vi "Target.vi"() -> ()   [LabVIEW 2013]
uses:
  shared/iRobot Sensor Display.ctl
  Statechart.lvsc/StatechartState.ctl
  Statechart.lvsc/State.ctl
  shared/Sensors.ctl
  iRobot/Sensor/Accelerometer.ctl
  iRobot/Sensor/Sensor Group 6.ctl
  iRobot/Sensor/Bumps + Wheel Drops.ctl
  iRobot/Sensor/Buttons.ctl
  iRobot/Sensor/Charging State.ctl
  iRobot/Sensor/Charging Sources Available.ctl
  iRobot/Sensor/OI Mode.ctl
  iRobot/Sensor/Cargo Bay Digital Inputs.ctl
  iRobot/Sensor/Low-Side Driver + Wheel Overcurrent.ctl
  Statechart.lvsc/CompanionDiagram.vi/42/SC Main.vi
  Statechart.lvsc/CompanionDiagram.vi/42/Upd State.vi
  Statechart.lvsc/CompanionDiagram.vi/42/Trans Graph0.vi
  Statechart.lvsc/CompanionDiagram.vi/42/EnterGraphCore.vi
  <vilib>/myRIO/Common/Instrument Driver Framework/myRIO v1.0/UART/vis/myRIO v1.0 Close UART.vi
  Statechart.lvsc/CompanionDiagram.vi/42/Trans Graph1.vi
  Statechart.lvsc/CompanionDiagram.vi/42/Trans Graph2.vi
  <vilib>/myRIO/Common/Instrument Driver Framework/myRIO v1.0/myRIO v1.1 Open.vi
  Statechart.lvsc/CompanionDiagram.vi
  shared/Wrap Angle.vi
  <vilib>/myRIO/Common/Instrument Driver Framework/Utilities/vis/FPGA Ref Manager.vi
  <vilib>/myRIO/Common/Instrument Driver Framework/myRIO v1.0/myRIO v1.0 Reset FPGA.vi
  Statechart.lvsc/Trigger.ctl
  <vilib>/Statechart/Infrastructure/RTStatechart/RunTime SCN.xnode
  Statechart.lvsc/Inputs.ctl
  Statechart.lvsc/Outputs.ctl
  Statechart.lvsc
  <vilib>/myRIO/Instrument Drivers/Utilities/Utilities.lvlib
panel:
  in  "Tab Control":T1(tab)
  out "iRobot Sensors (graphical)":T2 {"Right Wheel (mm/s)" scale=-500.0..500.0; "Left Wheel (mm/s)" scale=-500.0..500.0}
  out "Active States":T4
  out "error out":errorcluster
  in  "stop":bool
  out "Target Running":bool
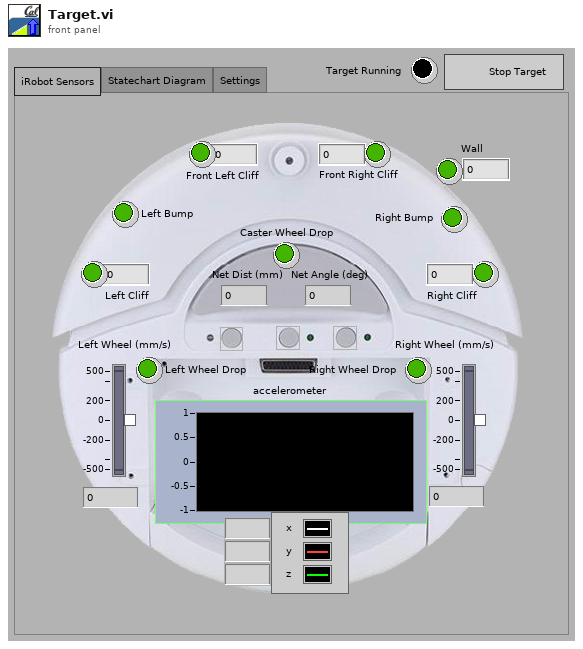
[diagram p1: front panel]
types:
  T1 = enum32{"iRobot Sensors", "Statechart Diagram", "Settings"}
  T2 = typedef "iRobot Sensor Display.ctl" = cluster{"Caster Wheel Drop":bool, "Left Wheel Drop":bool, "Right Wheel Drop":bool, "Left Bump":bool, "Right Bump":bool, "Left Cliff":bool, "Front Left Cliff":bool, "Front Right Cliff":bool, "Right Cliff":bool, "Wall":bool, "Net Dist (mm)":i32, "Net Angle (deg)":i32, "Wall":u16, "Left Cliff":u16, "Front Left Cliff":u16, "Front Right Cliff":u16, "Right Cliff":u16, "Left Wheel (mm/s)":i16, "Right Wheel (mm/s)":i16, "accelerometer":T3}
  T3 = typedef "Accelerometer.ctl" = cluster{"x axis (g)":dbl, "y axis (g)":dbl, "z axis (g)":dbl}
  T4 = typedef "Statechart.lvsc/StatechartState.ctl" = T5[]
  T5 = typedef "Statechart.lvsc/State.ctl" = enum16{"NI.SC.Initial", "NI.SC.History", "NI.SC.ShallowHistory", "NI.SC.Terminal", "Pause", "Run", "Pause\\Detect Play Button\\Pause;\nWait for\nbutton\nrelease", "Pause\\Detect Play Button\\Unpause;\nwait for\nbutton release", "Pause\\Detect Play Button\\Unpause;\nwait for\nbutton press", "Run\\Run Mode\\Turn", "Run\\Run Mode\\Drive"}
  T6 = typedef "iRobot UART Port Type.ctl" = refnum<visa-resource-name>
  T7 = typedef "Sensors.ctl" = cluster{"net distance (mm)":i32, "net angle (deg)":i32, "accelerometer":T3, "iRobot Sensors":T8, "Is Simulator?":bool}
  T8 = typedef "Sensor Group 6.ctl" = cluster{"Bumps + Wheel Drops":T9, "Wall":bool, "Cliff Left":bool, "Cliff Front Left":bool, "Cliff Front Right":bool, "Cliff Right":bool, "Wall Signal":u16, "Cliff Left Signal":u16, "Cliff Front Left Signal":u16, "Cliff Front Right Signal":u16, "Cliff Right Signal":u16, "Buttons":T10, "Virtual Wall":bool, "# Stream Packets":u8, "Requested Velocity (mm/s)":i16, "Requested Radius (mm)":i16, "Requested Right Wheel Velocity (mm/s)":i16, "Requested Left Wheel Velocity (mm/s)":i16, "Distance (mm)":i32, "Angle (deg)":i32, "Song Playing":bool, "Song Number":u8, "Charging State":T11, "Voltage (mV)":u16, "Current (mA)":i16, "Battery Temperature (deg C)":i8, "Battery Charge (mAh)":u16, "Battery Capacity (mAh)":u16, "Charging Sources":T12, "OI Mode":T13, "Digital Inputs":T14, "Drivers & Wheel Overcurrent":T15, "Analog Signal":u16, "Infrared":u8}
  T9 = typedef "Bumps + Wheel Drops.ctl" = cluster{"Wheeldrop Caster":bool, "Wheeldrop Left":bool, "Wheeldrop Right":bool, "Bump Left":bool, "Bump Right":bool}
  T10 = typedef "Buttons.ctl" = cluster{"Advance":bool, "Play":bool}
  T11 = typedef "Charging State.ctl" = enum16{"Not Charging", "Reconditioning Charging", "Full Charging", "Trickle Charging", "Waiting", "Charging Fault Condition"}
  T12 = typedef "Charging Sources Available.ctl" = cluster{"Internal Charger":bool, "Home Base":bool}
  T13 = typedef "OI Mode.ctl" = enum16{"Off", "Passive", "Safe", "Full"}
  T14 = typedef "Cargo Bay Digital Inputs.ctl" = cluster{"Digital Input 0":bool, "Digital Input 1":bool, "Digital Input 2":bool, "Digital Input 3":bool, "Device Detect":bool}
  T15 = typedef "Low-Side Driver + Wheel Overcurrent.ctl" = cluster{"Low-Side Driver 0":bool, "Low-Side Driver 1":bool, "Low-Side Driver 2":bool, "Left Wheel":bool, "Right Wheel":bool}
  T16 = typedef "Statechart.lvsc/Outputs.ctl" = cluster{"Left Wheel Speed (mm/s)":i16, "Right Wheel Speed (mm/s)":i16}
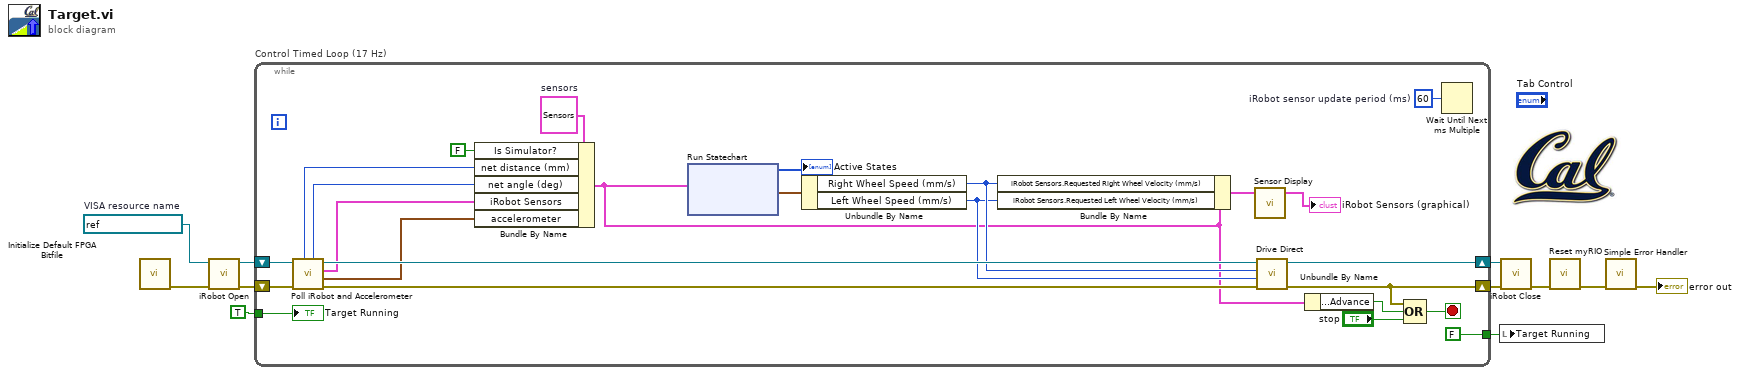
[diagram p0: block diagram]
diagram:
  w5 = refnum<visa-resource-name> "ASRL1::INSTR"  # VISA resource name
  n1 = call <vilib>:"Initialize Default FPGA Bitfile.vi"() -> ("error out"=w3:errorcluster)  [unwired: 11 in]
  n2 = call "iRobot Open.vi"("error in (no error)"=w3, "UART port in"=w5) -> ("error out"=w10:errorcluster, "UART port out"=w9:T6)  [unwired: 8 in]
  n3 = while "Control Timed Loop (17 Hz)" {
    shift-right: [w36] -> w11
    shift-left: w9 -> [w32]
    shift-right: [w16] -> w6
    shift-left: w10 -> [w31]
    tunnel: TRUE ("stop") -> [w26]
    tunnel: [FALSE ("stop")] -> w7
    stop <- w35 stop-if-true
    w18 = T7 {"net distance (mm)"=0, "net angle (deg)"=0, "accelerometer"={"x axis (g)"=0.0, "y axis (g)"=0.0, "z axis (g)"=0.0}, "iRobot Sensors"={"Bumps + Wheel Drops"={"Wheeldrop Caster"=FALSE, "Wheeldrop Left"=FALSE, "Wheeldrop Right"=FALSE, "Bump Left"=FALSE, "Bump Right"=FALSE}, "Wall"=FALSE, "Cliff Left"=FALSE, "Cliff Front Left"=FALSE, "Cliff Front Right"=FALSE, "Cliff Right"=FALSE, "Wall Signal"=0, "Cliff Left Signal"=0, "Cliff Front Left Signal"=0, "Cliff Front Right Signal"=0, "Cliff Right Signal"=0, "Buttons"={"Advance"=FALSE, "Play"=FALSE}, "Virtual Wall"=FALSE, "# Stream Packets"=0, "Requested Velocity (mm/s)"=0, "Requested Radius (mm)"=0, "Requested Right Wheel Velocity (mm/s)"=0, "Requested Left Wheel Velocity (mm/s)"=0, "Distance (mm)"=0, "Angle (deg)"=0, "Song Playing"=FALSE, "Song Number"=0, "Charging State"=enum."Not Charging", "Voltage (mV)"=0, "Current (mA)"=0, "Battery Temperature (deg C)"=0, "Battery Charge (mAh)"=0, "Battery Capacity (mAh)"=0, "Charging Sources"={"Internal Charger"=FALSE, "Home Base"=FALSE}, "OI Mode"=enum."Off", "Digital Inputs"={"Digital Input 0"=FALSE, "Digital Input 1"=FALSE, "Digital Input 2"=FALSE, "Digital Input 3"=FALSE, "Device Detect"=FALSE}, "Drivers & Wheel Overcurrent"={"Low-Side Driver 0"=FALSE, "Low-Side Driver 1"=FALSE, "Low-Side Driver 2"=FALSE, "Left Wheel"=FALSE, "Right Wheel"=FALSE}, "Analog Signal"=0, "Infrared"=255}, "Is Simulator?"=FALSE}  # sensors
    w20 = u32 60  # iRobot sensor update period (ms)
    n4 = call "Poll iRobot and Accelerometer.vi"("error in"=w31, "UART port in"=w32) -> ("error out"=w30:errorcluster, "Acceleration (g)"=w21:T3, "iRobot SensorGroup6"=w24:T8, "UART port out"=w29:T6, "net angle (deg)"=w27:i32, "net distance (mm)"=w28:i32)  [unwired: 4 in]
    n5 = Bundle By Name(cluster=w18, "Is Simulator?"=FALSE, "net distance (mm)"=w28, "net angle (deg)"=w27, "iRobot Sensors"=w24, "accelerometer"=w21) -> (w12:T7)
    n6 = xnode "Run Statechart"("Inputs"=w12) -> ("Outputs"=w34:T16, "Active States"=→"Active States":T4)  [unwired: 2 in, 1 out]
    n7 = Unbundle By Name(w34) -> ("Right Wheel Speed (mm/s)"=w15:i16, "Left Wheel Speed (mm/s)"=w14:i16)
    n8 = Bundle By Name(cluster=w12, "iRobot Sensors.Requested Right Wheel Velocity (mm/s)"=w15, "iRobot Sensors.Requested Left Wheel Velocity (mm/s)"=w14) -> (w13:T7)
    n9 = call "Sensor Display.vi"("sensors"=w13) -> ("irobot sensor display"=→"iRobot Sensors (graphical)":T2)  [unwired: 4 in]
    n10 = call "Drive Direct.vi"("error in"=w30, "Left Wheel Velocity (mm/s)"=w14, "Right Wheel Velocity (mm/s)"=w15, "UART port in"=w29) -> ("error out"=w16:errorcluster, "UART port out"=w36:T6)  [unwired: 6 in]
    n11 = Unbundle By Name(w12) -> ("iRobot Sensors.Buttons.Advance"=w22:bool)
    n12 = Compound Arithmetic op=OR(w16, w22, "stop") -> (w35:bool)
    n13 = Wait Until Next ms Multiple(millisecond multiple=w20) -> ()  [unwired: 1 out]
    "Target Running" <- w26
  }
  n14 = local write "Target Running"(w7) -> ()
  n15 = call "iRobot Close.vi"("error in"=w6, "UART port in"=w11) -> ("error out"=w1:errorcluster)  [unwired: 9 in]
  n16 = call <vilib>:"Reset myRIO.vi"("error in (no error)"=w1) -> ("error out"=w4:errorcluster)  [unwired: 10 in]
  n17 = call <vilib>:"Simple Error Handler.vi"("error in (no error)"=w4) -> ("error out"=→"error out":errorcluster)  [unwired: 4 in, 4 out]
